vi "client.new.vi"(7 "base_url":string, 8 "error in":errorcluster, 10 "workspace_rid":string, 11 "token":string) -> (0 "error out":errorcluster, 3 "Client out":refnum<class "Client.lvclass">)   [LabVIEW 2020, in "Client.lvclass"]
doc: "Releases the handle and its associated resources, closing the connection."
uses:
  Client.lvclass
  Client.lvclass/Client.ctl
  client.lvlib
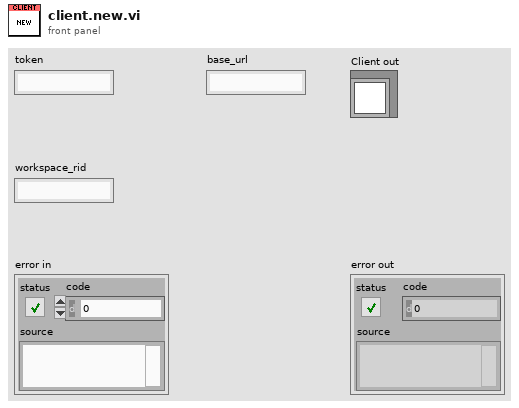
[diagram p1: front panel]
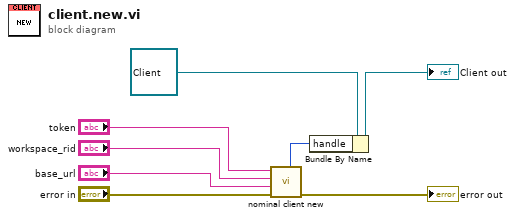
[diagram p0: block diagram]
diagram:
  n1 = call "nominal client new.vi"("error in (no error)"="error in", "base_url"="base_url", "workspace_rid"="workspace_rid", "token"="token") -> ("error out"=→"error out":errorcluster, "out_client out"=w8:i32)  [unwired: 5 in, 1 out]
  n2 = Bundle By Name(cluster=refnum<class "Client.lvclass"> refnum ("Client out"), "handle"=w8) -> (→"Client out":refnum<class "Client.lvclass">)
